vi "Write I.vi"(8 "error in (no error)":errorcluster, 10 "I":sgl, 11 "Update PID CMD in":refnum<class "Update PID CMD.lvclass">) -> (0 "error out":errorcluster, 3 "Update PID CMD out":refnum<class "Update PID CMD.lvclass">)   [LabVIEW 2014, in "Humidifier Lib.lvlib" / "Update PID CMD.lvclass"]
uses:
  Update PID CMD.lvclass
  Update PID CMD.lvclass/Update PID CMD.ctl
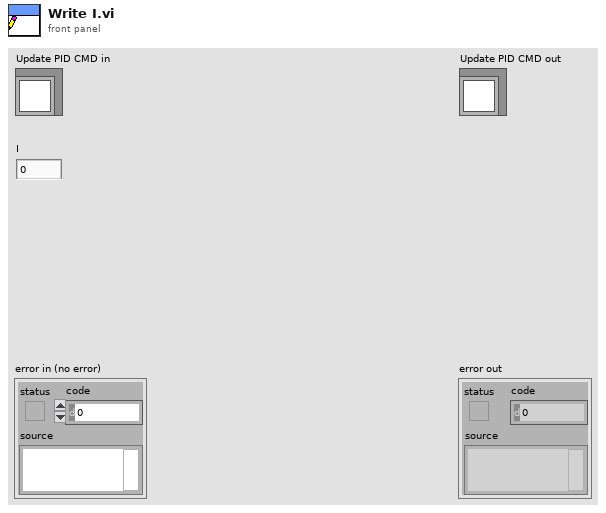
[diagram p1: front panel]
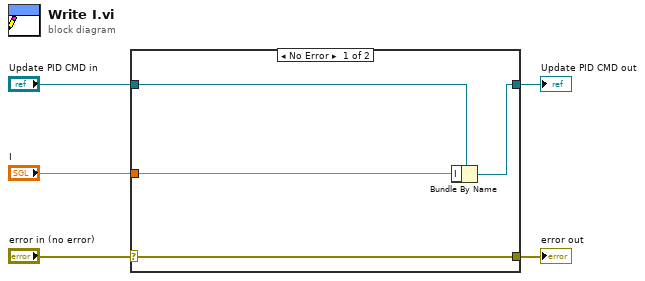
[diagram p0: block diagram]
diagram:
  n1 = case shown="No Error" "error in (no error)" {
    selector: "error in (no error)" -> [w9 w10]
    tunnel: [w9 w10] -> w4
    tunnel: [w7 w11] -> w2
    tunnel: "Update PID CMD in" -> [w8 w11]
    tunnel: "I" -> [w6 _]
    frame No Error {
      n2 = Bundle By Name(cluster=w8, "I"=w6) -> (w7:refnum<class "Update PID CMD.lvclass">)
    }
    frame Error {
    }
  }
  "error out" <- w4
  "Update PID CMD out" <- w2
